vi "Codebar Processing.vi"(5 "ROI Descriptor":T1={"Global Rectangle"=[10, 10, 1616, 1190], "Contours"=[{"ID"=enum."External", "Type"=12, "Coordinates"=[10, 10, 1616, 1190, 0]}]} {"Contours"."Type" items=["No Selection", "Point", "Line", "Rectangle", "Oval", "Polygon", "Freehand Region", "Annulus", "Unused2", "Unused3", "Broken Line", "Freehand Line", "Rotated Rectangle"]}, 8 "error in":errorcluster, 11 "Image In":T3) -> (0 "error out":errorcluster, 2 "Barcodes (Barcode Reader 1)":T2(array[cluster]) {"Confidence Level" format="%.2f"; "Barcode Type" items=["Reserved", "Codabar", "Code 39", "Code 93", "Code 128", "EAN 8", "EAN 13", "Interleaved 2 of 5", "MSI", "UPCA", "Pharmacode", "RSS Limited"]; "Bounding Box"."y" format="%.2f"; "Bounding Box"."x" format="%.2f"}, 3 "Image Out":T3)   [LabVIEW 2018]
uses:
  <vilib>/vision/Image Controls.llb/IMAQ Image.ctl
  <vilib>/vision/NI_Vision_Development_Module.lvlib
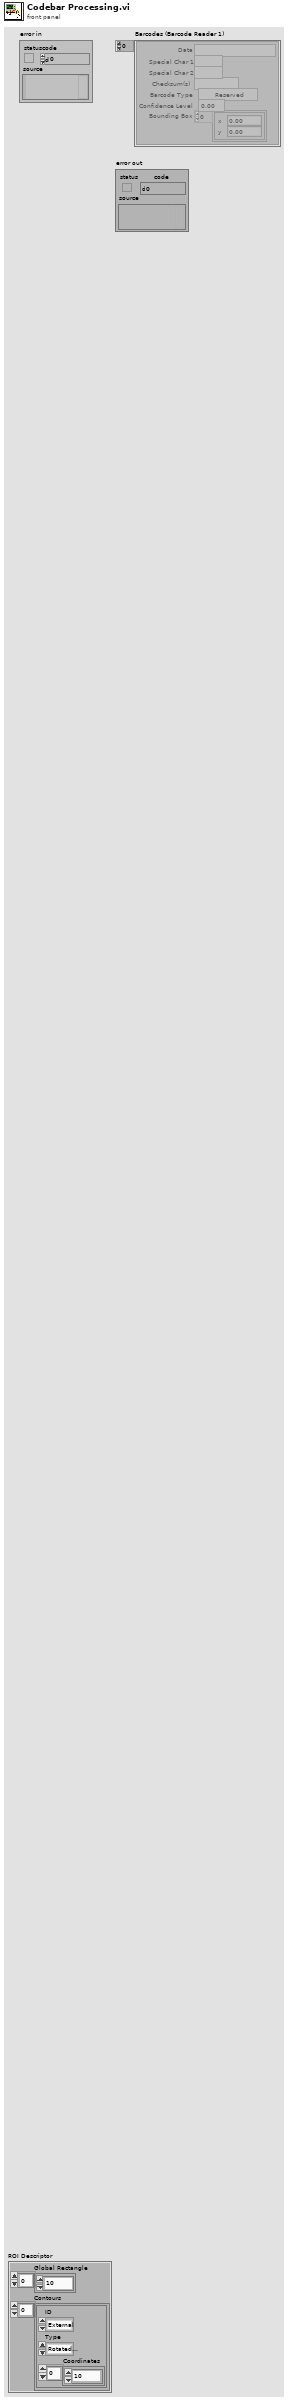
[diagram p1: front panel]
types:
  T1 = cluster{"Global Rectangle":i32[], "Contours":cluster{"ID":enum32{"External", "Internal"}, "Type":u32, "Coordinates":i32[]}[]}
  T2 = cluster{"Data":string, "Special Char 1":string, "Special Char 2":string, "Checksum(s)":string, "Barcode Type":u32, "Confidence Level":sgl, "Bounding Box":cluster{"x":sgl, "y":sgl}[]}[]
  T3 = typedef "IMAQ Image.ctl" = refnum<image>
  T4 = cluster{"Calculate Grading Report":bool, "Scan Width ":i32}
  T5 = cluster{"Min Bar Width":u32, "Min Edge Strength":u32, "Min Bars":u32, "Skip Location Search?":bool}
  T6 = cluster{"histogram":u32[], "Minimal Value":sgl, "Maximal Value":sgl, "Starting Value":sgl, "Interval Width":sgl, "Mean Value":sgl, "Standard  Variation":sgl, "Area (pixels)":i32}
  T7 = typedef "Image Type" = u32
  T8 = cluster{"Overall Grade":string, "Edge Determination Grade":string, "Minimum Reflectance Grade":string, "Minimum Edge Contrast Grade":string, "Symbol Contrast Grade":string, "Modulation Grade":string, "Defects Grade":string, "Decode Grade":string, "Decodability Grade":string, "Quiet Zone":string}[]
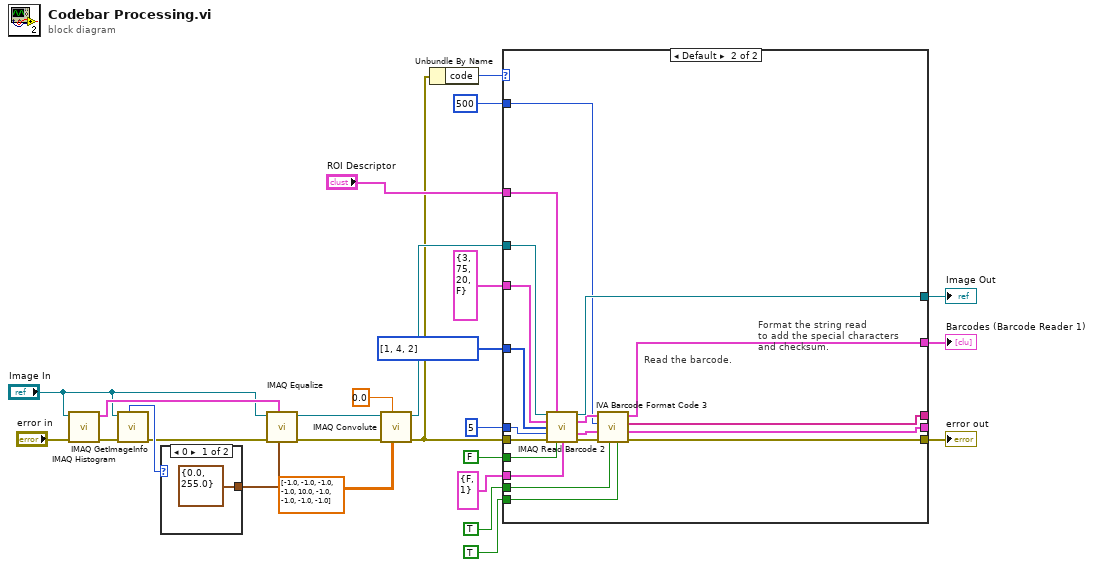
[diagram p0: block diagram]
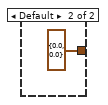
[diagram p3: hidden frame]
diagram:
  w6 = u32[] [1, 4, 2] items=["Reserved", "Codabar", "Code 39", "Code 93", "Code 128", "EAN 8", "EAN 13", "Interleaved 2 of 5", "MSI", "UPCA", "Pharmacode", "RSS Limited"] ("Barcode Types To Search")
  n1 = call "IMAQ Histogram"("error in (no error)"="error in", "Image"="Image In") -> ("error out"=w22:errorcluster, "Histogram Report"=w26:T6)  [unwired: 3 in, 5 out]
  n2 = call "IMAQ GetImageInfo"("error in (no error)"=w22, "Image"="Image In") -> ("error out"=w21:errorcluster, "Image Type"=w24:T7)  [unwired: 8 out]
  n3 = case shown="0" w24 {
    tunnel: [cluster{"Minimum":sgl, "Maximum":sgl} {"Minimum"=0.0, "Maximum"=255.0} ("Range") cluster{"Minimum":sgl, "Maximum":sgl} {"Minimum"=0.0, "Maximum"=0.0} ("Range")] -> w20
    frame 0 {
    }
    frame Default {
    }
  }
  n4 = call "IMAQ Equalize"("Range"=w20, "Histogram Report"=w26, "error in (no error)"=w21, "Image Src"="Image In") -> ("error out"=w17:errorcluster, "Image Dst Out"=w18:T3)  [unwired: 2 in, 4 out]
  n5 = call "IMAQ Convolute"("Kernel"=sgl[][] [[-1.0, -1.0, -1.0], [-1.0, 10.0, -1.0], [-1.0, -1.0, -1.0]], "Divider (kernel sum)"=sgl 0.0 ("Divider"), "error in (no error)"=w17, "Image Src"=w18) -> ("error out"=w9:errorcluster, "Image Dst Out"=w12:T3)  [unwired: 3 in, 3 out]
  n6 = Unbundle By Name(w9) -> ("code"=w8:i32)
  n7 = case shown="Default" w8 {
    tunnel: w9 -> [w29 w46]
    tunnel: FALSE ("Validate") -> [_ w42]
    tunnel: TRUE ("Add Special Characters") -> [_ w34]
    tunnel: TRUE ("Add Checksum") -> [_ w35]
    tunnel: w12 -> [w30 w49]
    tunnel: "ROI Descriptor" -> [_ w47]
    tunnel: [w30 w48] -> w10
    tunnel: T5 {"Min Bar Width"=3, "Min Edge Strength"=75, "Min Bars"=20, "Skip Location Search?"=FALSE} ("Barcode Search Options") -> [_ w45]
    tunnel: w6 -> [_ w44]
    tunnel: u32 5 ("Num of Required Barcodes") -> [_ w43]
    tunnel: u16 500 ("Minimum Score") -> [_ w40]
    tunnel: [w29 w38] -> w3
    tunnel: [_ w37] -> w2
    tunnel: [_ w36] -> _
    tunnel: [_ w32] -> _
    tunnel: T4 {"Calculate Grading Report"=FALSE, "Scan Width "=1} ("Barcode Grading Options") -> [_ w31]
    frame -1074396199, -1074396198 {
      # "Discard Coordinate System Error"
    }
    frame Default {
      # "Format the string read\nto add the special characters\nand checksum."
      # "Read the barcode."
      n8 = call "IMAQ Read Barcode 2"("Image"=w49, "ROI Descriptor"=w47, "Barcode Search Options"=w45, "Barcode Types To Search"=w44, "Num of Required Barcodes"=w43, "error in (no error)"=w46, "Validate"=w42, "Barcode Grading Options"=w31) -> ("Image (duplicate)"=w48:T3, "Barcodes"=w41:T2, "Barcode ANSI/CEN/ISO Grading Report"=w33:T8, "error out"=w39:errorcluster)  [unwired: 3 in, 1 out]
      n9 = call <vilib>:"IVA Barcode Format Code 3.vi"("Add Checksum"=w35, "Add Special Characters"=w34, "error in (no error)"=w39, "Barcode Grading Report in"=w33, "Minimum Score"=w40, "Barcodes in"=w41) -> ("error out"=w38:errorcluster, "Barcode Grading Report out"=w32:T8, "Complete Data"=w36:string[], "Barcodes out"=w37:T2)  [unwired: 2 in]
    }
  }
  "error out" <- w3
  "Image Out" <- w10
  "Barcodes (Barcode Reader 1)" <- w2
